vi "))Channel.vi"(0 "EnclaveChannel in":T2, 2 "This VI in":refnum<vi>, 7 "Operation":T1) -> (3 "This VI out":refnum<vi>, 4 "EnclaveChannel out":T2)   [LabVIEW 2022 SP3, in "Enclave.lvlib"]
uses:
  Enclave.lvlib
  ))Channel.ctl
  Element.ctl
  Operation.ctl
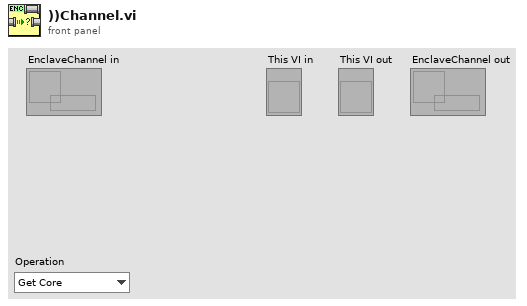
[diagram p1: front panel]
types:
  T1 = typedef "Enclave.lvlib/Operation.ctl" = enum16{"Get Core", "Init", "Close"}
  T2 = typedef "Enclave.lvlib/))Channel.ctl" = refnum<queue>
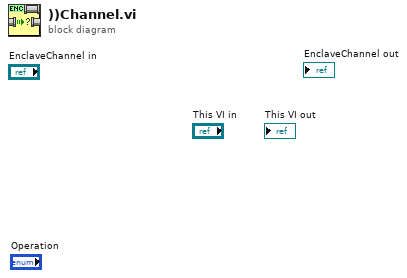
[diagram p0: block diagram]
diagram:
